vi "CLD 4 Event Structure Timer Solution.vi"() -> ()   [LabVIEW 2009]
doc: "CLD-Zusatzaufgabe 4\n\nDieses VI veranschaulicht die Verwendung des Timeout-Anschlusses der Ereignisstruktur in Verbindung mit der Verarbeitung von Werten.\n\nObwohl das Frontpanel den Timern in vorherigen CLD-Übungen ähnelt, ist der Timer nicht zum Messen der Zeit geeignet. Beim Messen der Zeit wird nur die Anzahl der Timeouts gezählt und mit jedem aufgetretenen Timeout wird eine Zeit assoziiert.\n\nWenn noch andere Ereignisse eintreten würden, wäre das Timing nicht konsekutiv. Die Verwendung des Timeout-Anschlusses einer Ereignisstruktur zum eigentlichen Verarbeiten des Timings ist nur dann ein zuverlässige Methode, wenn auch Inaktivität aufgezeichnet wird."
panel:
  out "Verstrichene Zeit":dbl
  out "Fehler (Ausgang)":T1
  in  "Fehler (Eingang)":T1
  out "Bit 4":bool
  out "Bit 3":bool
  out "Bit 2":bool
  out "Bit 1":bool
  out "Zeit ist verstrichen":bool
  in  "Autom. zurücksetzen":bool
  in  "Zurücksetzen-Schaltfläche":bool
  in  "VI anhalten":bool
  in  "Zielzeit (s)":dbl
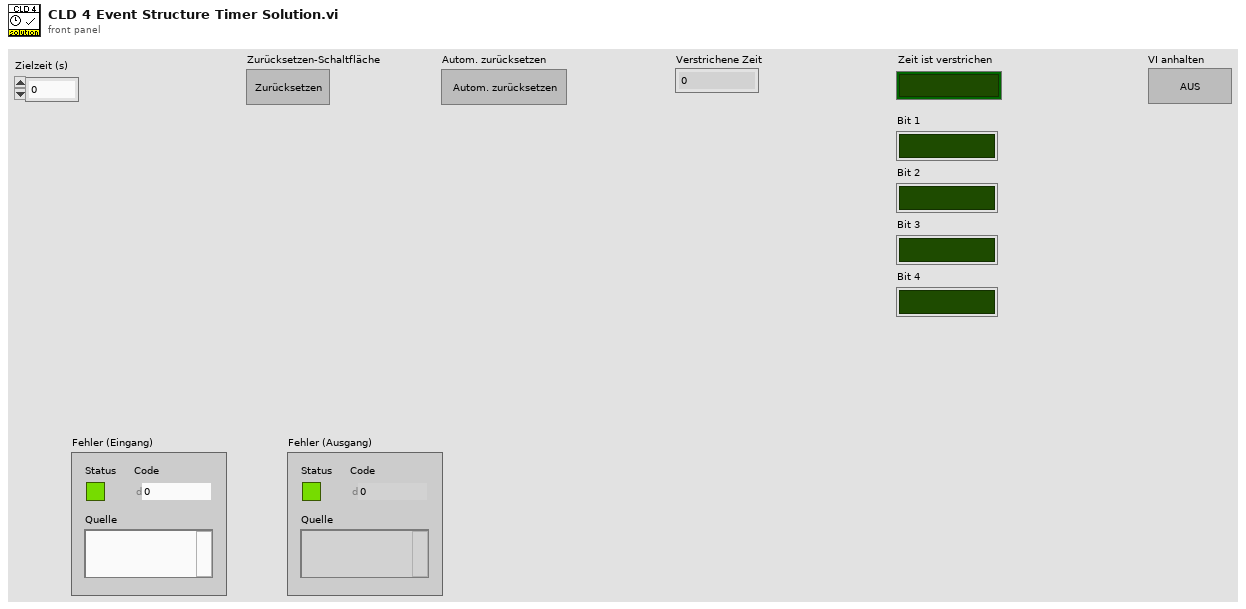
[diagram p1: front panel]
types:
  T1 = cluster{"Status":bool, "Code":i32, "Quelle":string}
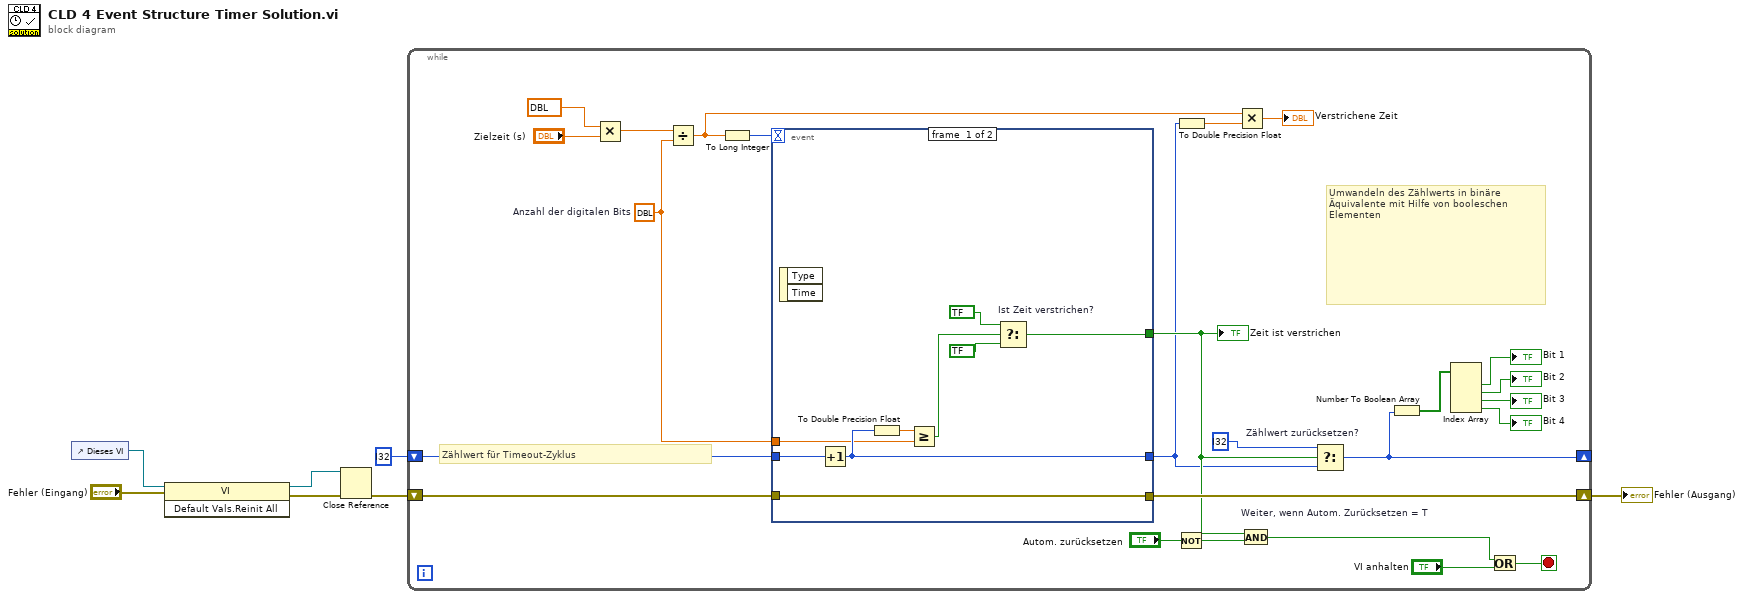
[diagram p0: block diagram]
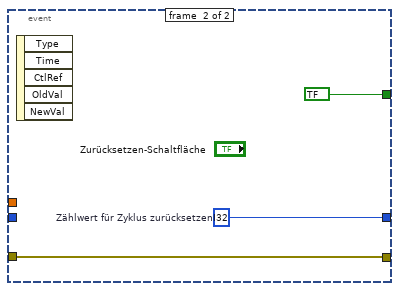
[diagram p2: hidden frame]
diagram:
  n1 = control-ref of="Dieses VI"() -> (w3:refnum<vi>)
  n2 = invoke on="Invoke Node" class="VI" method="Default Vals.Reinit All"(reference=w3, error in="Fehler (Eingang)") -> (reference out=w1:refnum<vi>, error out=w4:errorcluster)  [unwired: 1 in, 1 out]
  n3 = Close Reference(reference=w1, error in (no error)=w4) -> (error out=w2:errorcluster)
  n4 = while {
    shift-right: [w12] -> _
    shift-left: i32 ? -> [w31]
    shift-right: [w24] -> w5
    shift-left: w2 -> [w25]
    stop <- w20 stop-if-true
    w11 = dbl ?  # Anzahl der digitalen Bits
    # "Umwandeln des Zählwerts in binäre Äquivalente mit Hilfe von booleschen Elementen"
    # "Zählwert für Timeout-Zyklus"
    n5 = Multiply(x=dbl ?, y="Zielzeit (s)") -> (x*y=w22:dbl)
    n6 = Divide(x=w22, y=w11) -> (x/y=w18:dbl)
    n7 = To Long Integer(number=w18) -> (32bit integer=w8:i32)
    n8 = event shown="[1] \"Zurücksetzen-Schaltfläche\": Value Change" {
      selector: _ -> [_ _]
      dyn-events: _ -> [_ _]
      timeout: w8 -> [_ _]
      tunnel: [w35 w43] -> w13
      tunnel: w31 -> [w41 _]
      tunnel: [w37 bool ?] -> w15
      tunnel: w25 -> [w36 w42]
      tunnel: [w36 w42] -> w24
      tunnel: w11 -> [w34 _]
      event #0 {
        n9 = event-data() -> ()  [unwired: 1 in, 2 out]
        n10 = Increment(x=w41) -> (x+1=w35:i32)
        n11 = To Double Precision Float(number=w35) -> (double precision float=w33:dbl)
        n12 = Greater Or Equal?(x=w33, y=w34) -> (x >= y?=w40:bool)
        n13 = Select "Ist Zeit verstrichen?"(t=bool ?, s=w40, f=bool ?) -> (s? t:f=w37:bool)
      }
      event #1 {
        w43 = i32 ?  # Zählwert für Zyklus zurücksetzen
        n14 = event-data() -> ()  [unwired: 1 in, 5 out]
      }
    }
    "Zeit ist verstrichen" <- w15
    n15 = Not(x="Autom. zurücksetzen") -> (.not. x?=w16:bool)
    n16 = To Double Precision Float(number=w13) -> (double precision float=w10:dbl)
    n17 = Multiply(x=w18, y=w10) -> (x*y=→"Verstrichene Zeit":dbl)
    n18 = And "Weiter, wenn Autom. Zurücksetzen = T"(x=w15, y=w16) -> (x .and. y?=w19:bool)
    n19 = Select "Zählwert zurücksetzen?"(t=i32 ?, s=w15, f=w13) -> (s? t:f=w12:i32)
    n20 = Number To Boolean Array(number=w12) -> (Boolean array=w30:bool[])
    n21 = Index Array(array=w30) -> (element #1=→"Bit 1":bool, element #2=→"Bit 2":bool, element #3=→"Bit 3":bool, element #4=→"Bit 4":bool)  [unwired: 4 in]
    n22 = Or(x=w19, y="VI anhalten") -> (x .or. y?=w20:bool)
  }
  "Fehler (Ausgang)" <- w5
